vi "GetCellData.vi"(8 "error in (no error)":errorcluster, 9 "start column":i32, 10 "start row":i32, 11 "report in":refnum<class "NI_report.lvclass">) -> (0 "error out":errorcluster, 2 "data":string, 3 "report out":refnum<class "NI_report.lvclass">)   [LabVIEW 2012]
uses:
  <vilib>/Utility/NIReport.llb/NI_report.lvclass
  <vilib>/addons/_office/excel.llb/Excel Get Data (str).vi
  <vilib>/addons/_office/NI_ReportGenerationToolkit.lvlib
  <vilib>/Utility/NIReport.llb/Excel/NI_Excel.lvclass
panel:
  in  "start (0, 0)":cluster{"start row":i32, "start column":i32}
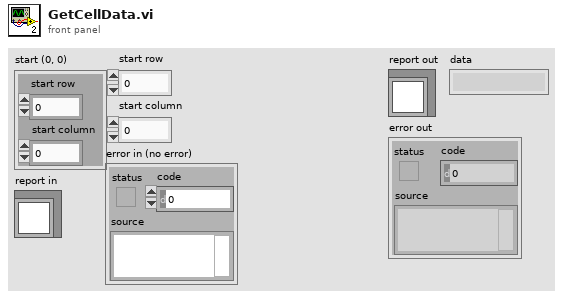
[diagram p1: front panel]
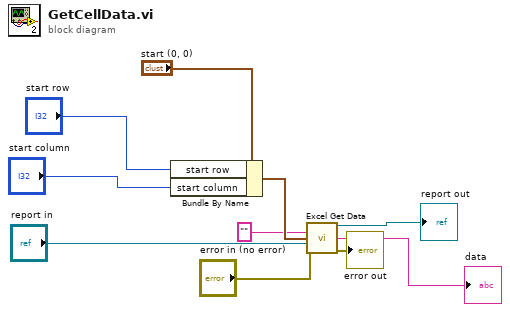
[diagram p0: block diagram]
diagram:
  n1 = Bundle By Name(cluster="start (0, 0)", "start row"="start row", "start column"="start column") -> (w10:cluster{"start row":i32, "start column":i32})
  n2 = call-poly <vilib>:"Excel Get Data.vi"("report in"="report in", "data type"="", "start (0, 0)"=w10, "error in (no error)"="error in (no error)") -> ("report out"=→"report out":refnum<class "NI_report.lvclass">, "data"=→"data":string, "error out"=→"error out":errorcluster)  [unwired: 9 in]
